vi "moveToJumperPosition-v02.vi"(0 "which manipulator":T3(ring), 1 "controls array in":refnum<vi>[](array[refnum]), 7 "Which Jumper Position to move to?":T1(ring), 9 "setStatus?":bool=TRUE, 11 "error in":errorcluster, 12 "common cluster":T2) -> (3 "control array out":refnum<vi>[](array[refnum]), 15 "error out":errorcluster)   [LabVIEW 2019]
uses:
  multipatch/controls/multipatch_common_controls_v4.ctl
  machine_vision/controls/transform_cluster_actuator.ctl
  machine_vision/coordinate model vis/transform_properties_actuators.ctl
  pipette cleaning/pressure box/cleaning_soft/controls/actuator_cluster.ctl
  pipette cleaning/pressure box/cleaning_soft/controls/actuator_type.ctl
  pipette cleaning/pressure box/cleaning_soft/controls/pressure_box_control.ctl
  pipette cleaning/pressure box/cleaning_soft/controls/pressure_box_type.ctl
  controls/NH_method.ctl
  controls/scope_motion.ctl
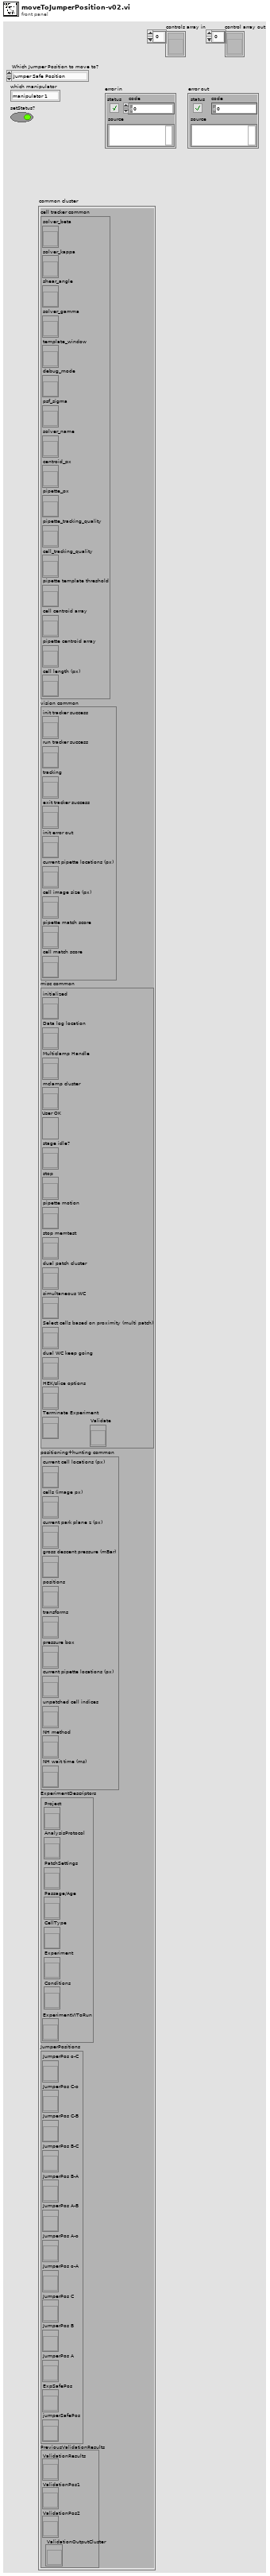
[diagram p1: front panel]
types:
  T1 = enum16{"Jumper Safe Position", "Experiment Safe Position", "Jumper Position A", "Jumper Position B", "Jumper Position C", "Jumper Position o-A", "Jumper Position A-o", "Jumper Position A-B", "Jumper Position B-A", "Jumper Position B-C", "Jumper Position C-B", "Jumper Position C-o", "Jumper Position o-C"}
  T2 = typedef "multipatch_common_controls_v4.ctl" = cluster{"cell tracker common":cluster{"solver_beta":refnum<vi>, "solver_kappa":refnum<vi>, "shear_angle":refnum<vi>, "solver_gamma":refnum<vi>, "template_window":refnum<vi>, "debug_mode":refnum<vi>, "psf_sigma":refnum<vi>, "solver_name":refnum<vi>, "centroid_px":refnum<vi>, "pipette_px":refnum<vi>, "pipette_tracking_quality":refnum<vi>, "cell_tracking_quality":refnum<vi>, "pipette template threshold":refnum<vi>, "cell centroid array":refnum<vi>, "pipette centroid array":refnum<vi>, "cell length (px)":refnum<vi>}, "vision common":cluster{"init tracker success":refnum<vi>, "run tracker success":refnum<vi>, "tracking":refnum<vi>, "exit tracker success":refnum<vi>, "init error out":refnum<vi>, "current pipette locations (px)":refnum<vi>, "cell image size (px)":refnum<vi>, "pipette match score":refnum<vi>, "cell match score":refnum<vi>}, "misc common":cluster{"initialized":refnum<vi>, "Data log location":refnum<vi>, "Multiclamp Handle":refnum<vi>, "mclamp cluster":refnum<vi>, "User OK":refnum<vi>, "stage idle?":refnum<vi>, "stop":refnum<vi>, "pipette motion":refnum<vi>, "stop memtest":refnum<vi>, "dual patch cluster":refnum<vi>, "simultaneous WC":refnum<vi>, "Select cells based on proximity (multi patch)":refnum<vi>, "dual WC keep going":refnum<vi>, "HEK/slice options":refnum<vi>, "Terminate Experiment":refnum<vi>, "Validate":refnum<vi>}, "positioning+hunting common":cluster{"current cell locations (px)":refnum<vi>, "cells (image px)":refnum<vi>, "current park plane z (px)":refnum<vi>, "gross descent pressure (mBar)":refnum<vi>, "positions":refnum<vi>, "transforms":refnum<vi>, "pressure box":refnum<vi>, "current pipette locations (px)":refnum<vi>, "unpatched cell indices":refnum<vi>, "NH method":refnum<vi>, "NH wait time (ms)":refnum<vi>}, "ExperimentDescriptors":cluster{"Project":refnum<vi>, "AnalysisProtocol":refnum<vi>, "PatchSettings":refnum<vi>, "Passage/Age":refnum<vi>, "CellType":refnum<vi>, "Experiment":refnum<vi>, "Conditions":refnum<vi>, "ExperimentVIToRun":refnum<vi>}, "JumperPositions":cluster{"JumperPos o-C":refnum<vi>, "JumperPos C-o":refnum<vi>, "JumperPos C-B":refnum<vi>, "JumperPos B-C":refnum<vi>, "JumperPos B-A":refnum<vi>, "JumperPos A-B":refnum<vi>, "JumperPos A-o":refnum<vi>, "JumperPos o-A":refnum<vi>, "JumperPos C":refnum<vi>, "JumperPos B":refnum<vi>, "JumperPos A":refnum<vi>, "ExpSafePos":refnum<vi>, "jumperSafePos":refnum<vi>}, "PreviousValidationResults":cluster{"ValidationResults":refnum<vi>, "ValidationPos1":refnum<vi>, "ValidationPos2":refnum<vi>, "ValidationOutputCluster":refnum<vi>}}
  T3 = enum16{"manipulator 1", "manipulator 2", "manipulator 3", "manipulator 4"}
  T4 = cluster{"JumperPos o-C":refnum<vi>, "JumperPos C-o":refnum<vi>, "JumperPos C-B":refnum<vi>, "JumperPos B-C":refnum<vi>, "JumperPos B-A":refnum<vi>, "JumperPos A-B":refnum<vi>, "JumperPos A-o":refnum<vi>, "JumperPos o-A":refnum<vi>, "JumperPos C":refnum<vi>, "JumperPos B":refnum<vi>, "JumperPos A":refnum<vi>, "ExpSafePos":refnum<vi>, "jumperSafePos":refnum<vi>}
  T5 = typedef "pressure_box_control.ctl" = cluster{"Pressure box COM":refnum<visa-resource-name>, "pressure box type":T6, "High pos pressure (mBar)":dbl, "Low pos pressure (mBar)":dbl, "Vacuum pressure (mBar)":dbl, "calibration":enum16{"PA_vacPump", "PA_venturi", "Neuromatics", "ilyaRig", "mightenRig"}}
  T6 = typedef "pressure_box_type.ctl" = enum16{"Neuromatics", "ProportionAir", "Demo box", "N-ProportionAir"}
  T7 = cluster{"current stage pos (steps)":refnum<vi>, "current manip 1 pos (steps)":refnum<vi>, "current manip 2 pos (steps)":refnum<vi>, "current manip 3 pos (steps)":refnum<vi>, "current manip 4 pos (steps)":refnum<vi>}
  T8 = typedef "transform_cluster_actuator.ctl" = cluster{"s":refnum<vi>, "manip 1":refnum<vi>, "manip 2":refnum<vi>, "manip 3":refnum<vi>, "manip 4":refnum<vi>}
  T9 = typedef "scope_motion.ctl" = enum16{"superSlow", "fast", "slow", "find slice speed", "slow_dualPatch"}
  T10 = typedef "transform_properties_actuators.ctl" = cluster{"theta (deg)":dbl, "X sc factor (px/step)":dbl, "Y sc factor (px/step)":dbl, "zero loc (x,y,z)":dbl[], "flip y?":bool, "flip x?":bool, "gamma (deg)":dbl, "flip z?":bool, "Z sc factor (px/step)":dbl, "actuator":T11, "safe space (steps)":i32[]}
  T11 = typedef "actuator_cluster.ctl" = cluster{"Actuator COM":refnum<visa-resource-name>, "Actuator type":T12}
  T12 = typedef "actuator_type.ctl" = enum16{"Scientifica", "Sutter", "Demo", "Off"}
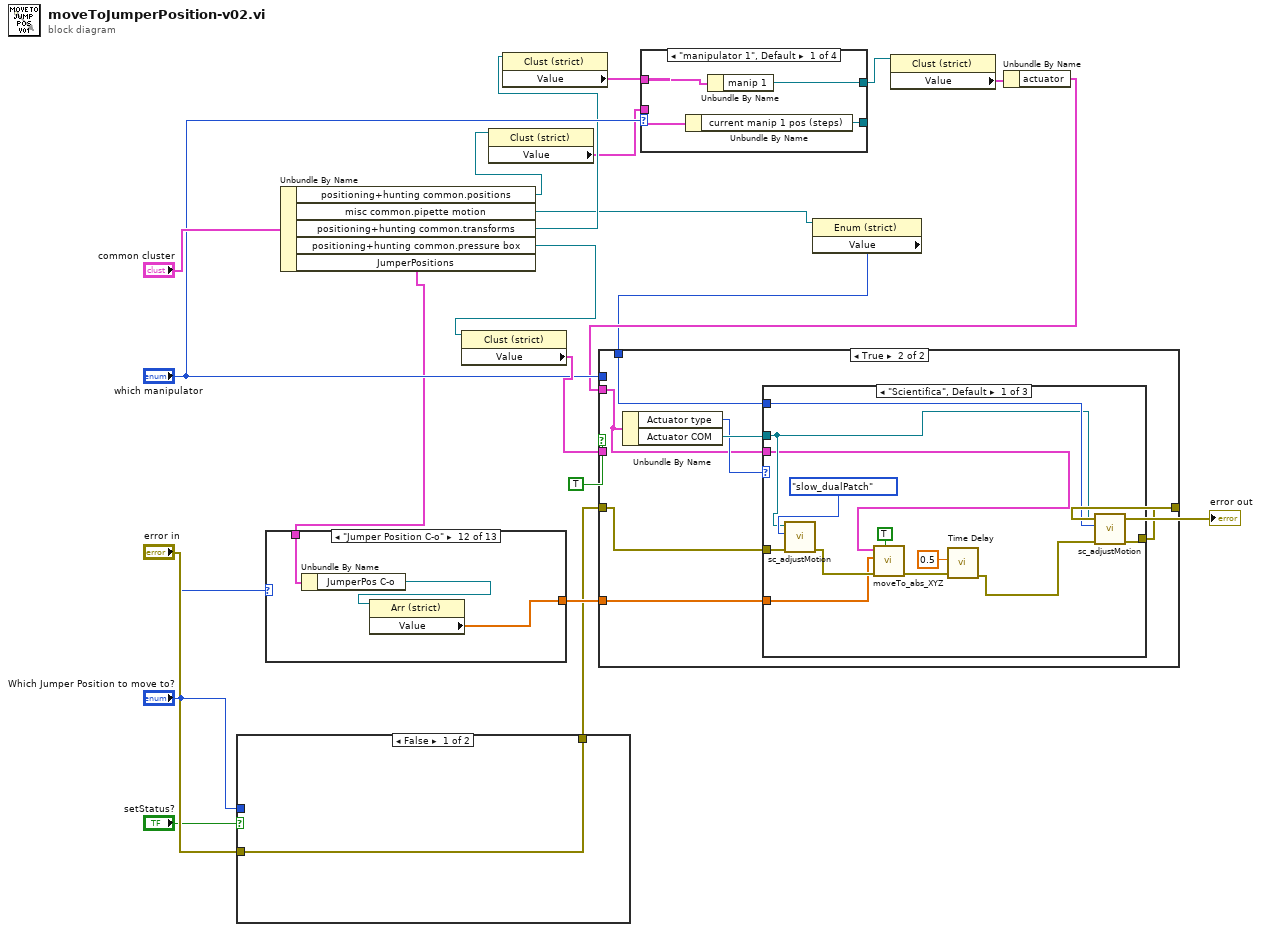
[diagram p0: block diagram]
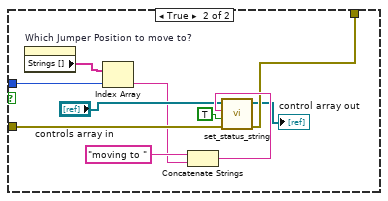
[diagram p2: hidden frame]
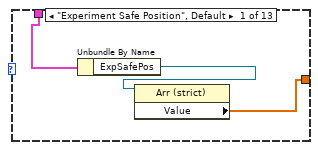
[diagram p3: hidden frame]
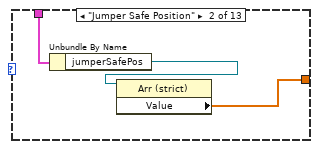
[diagram p4: hidden frame]
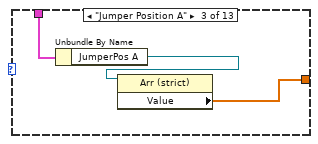
[diagram p5: hidden frame]
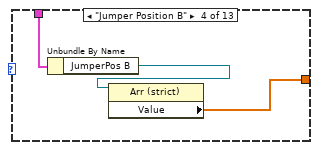
[diagram p6: hidden frame]
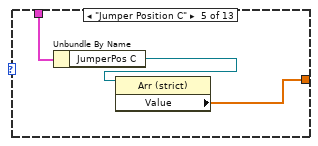
[diagram p7: hidden frame]
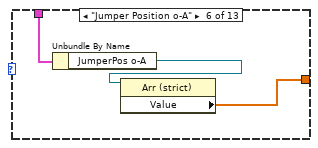
[diagram p8: hidden frame]
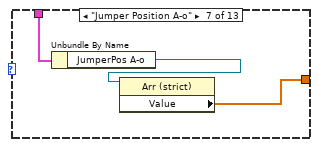
[diagram p9: hidden frame]
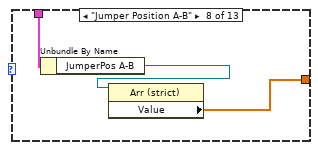
[diagram p10: hidden frame]
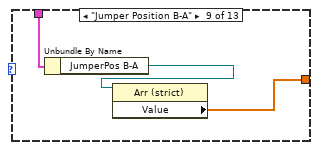
[diagram p11: hidden frame]
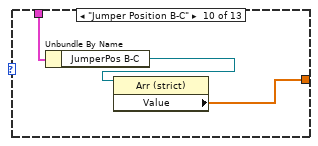
[diagram p12: hidden frame]
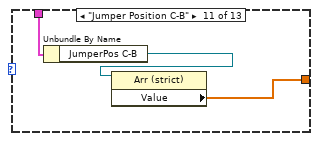
[diagram p13: hidden frame]
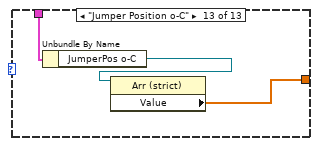
[diagram p14: hidden frame]
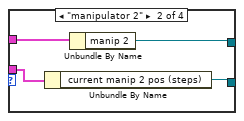
[diagram p15: hidden frame]
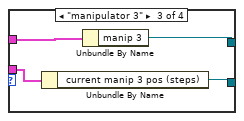
[diagram p16: hidden frame]
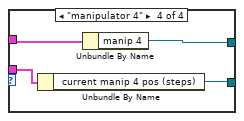
[diagram p17: hidden frame]
diagram:
  n1 = case shown="False" "setStatus?" {
    tunnel: "error in" -> [w22 w29]
    tunnel: [w22 w28] -> w3
    tunnel: "Which Jumper Position to move to?" -> [_ w24]
    frame False {
    }
    frame True {
      n2 = property on="Which Jumper Position to move to?" class="Enum (strict)"() -> ("Strings []"=w25:string[])  [unwired: 2 in, 2 out]
      n3 = Index Array(array=w25, index=w24) -> (element=w23:string)
      n4 = Concatenate Strings("moving to " ("string"), w23) -> (w31:string)
      n5 = call "set_status_string.vi"("error in"=w29, "new line?"=TRUE, "status string in"=w31, "controls array"="controls array in") -> ("error out"=w28:errorcluster, "controls array out"=→"control array out":refnum<vi>[])  [unwired: 6 in]
    }
  }
  n6 = Unbundle By Name("common cluster") -> ("positioning+hunting common.positions"=w6:refnum<vi>, "misc common.pipette motion"=w11:refnum<vi>, "positioning+hunting common.transforms"=w12:refnum<vi>, "positioning+hunting common.pressure box"=w20:refnum<vi>, "JumperPositions"=w5:T4)
  n7 = case shown="\"Jumper Position C-o\"" "Which Jumper Position to move to?" {
    tunnel: [w33 w36 w39 w42 w46 w49 w52 w55 w58 w61 w64 w67 w70] -> w7
    tunnel: w5 -> [w35 w37 w40 w43 w45 w48 w51 w54 w57 w60 w63 w66 w69]
    frame "Experiment Safe Position", Default {
      n8 = Unbundle By Name(w35) -> ("ExpSafePos"=w34:refnum<vi>)
      n9 = property class="Arr (strict)"(reference=w34) -> ("Value"=w33:dbl[])  [unwired: 1 in, 2 out]
    }
    frame "Jumper Safe Position" {
      n10 = Unbundle By Name(w37) -> ("jumperSafePos"=w38:refnum<vi>)
      n11 = property class="Arr (strict)"(reference=w38) -> ("Value"=w36:dbl[])  [unwired: 1 in, 2 out]
    }
    frame "Jumper Position A" {
      n12 = Unbundle By Name(w40) -> ("JumperPos A"=w41:refnum<vi>)
      n13 = property class="Arr (strict)"(reference=w41) -> ("Value"=w39:dbl[])  [unwired: 1 in, 2 out]
    }
    frame "Jumper Position B" {
      n14 = Unbundle By Name(w43) -> ("JumperPos B"=w44:refnum<vi>)
      n15 = property class="Arr (strict)"(reference=w44) -> ("Value"=w42:dbl[])  [unwired: 1 in, 2 out]
    }
    frame "Jumper Position C" {
      n16 = Unbundle By Name(w45) -> ("JumperPos C"=w47:refnum<vi>)
      n17 = property class="Arr (strict)"(reference=w47) -> ("Value"=w46:dbl[])  [unwired: 1 in, 2 out]
    }
    frame "Jumper Position o-A" {
      n18 = Unbundle By Name(w48) -> ("JumperPos o-A"=w50:refnum<vi>)
      n19 = property class="Arr (strict)"(reference=w50) -> ("Value"=w49:dbl[])  [unwired: 1 in, 2 out]
    }
    frame "Jumper Position A-o" {
      n20 = Unbundle By Name(w51) -> ("JumperPos A-o"=w53:refnum<vi>)
      n21 = property class="Arr (strict)"(reference=w53) -> ("Value"=w52:dbl[])  [unwired: 1 in, 2 out]
    }
    frame "Jumper Position A-B" {
      n22 = Unbundle By Name(w54) -> ("JumperPos A-B"=w56:refnum<vi>)
      n23 = property class="Arr (strict)"(reference=w56) -> ("Value"=w55:dbl[])  [unwired: 1 in, 2 out]
    }
    frame "Jumper Position B-A" {
      n24 = Unbundle By Name(w57) -> ("JumperPos B-A"=w59:refnum<vi>)
      n25 = property class="Arr (strict)"(reference=w59) -> ("Value"=w58:dbl[])  [unwired: 1 in, 2 out]
    }
    frame "Jumper Position B-C" {
      n26 = Unbundle By Name(w60) -> ("JumperPos B-C"=w62:refnum<vi>)
      n27 = property class="Arr (strict)"(reference=w62) -> ("Value"=w61:dbl[])  [unwired: 1 in, 2 out]
    }
    frame "Jumper Position C-B" {
      n28 = Unbundle By Name(w63) -> ("JumperPos C-B"=w65:refnum<vi>)
      n29 = property class="Arr (strict)"(reference=w65) -> ("Value"=w64:dbl[])  [unwired: 1 in, 2 out]
    }
    frame "Jumper Position C-o" {
      n30 = Unbundle By Name(w66) -> ("JumperPos C-o"=w68:refnum<vi>)
      n31 = property class="Arr (strict)"(reference=w68) -> ("Value"=w67:dbl[])  [unwired: 1 in, 2 out]
    }
    frame "Jumper Position o-C" {
      n32 = Unbundle By Name(w69) -> ("JumperPos o-C"=w71:refnum<vi>)
      n33 = property class="Arr (strict)"(reference=w71) -> ("Value"=w70:dbl[])  [unwired: 1 in, 2 out]
    }
  }
  n34 = property class="Clust (strict)"(reference=w20) -> ("Value"=w18:T5)  [unwired: 1 in, 2 out]
  n35 = property class="Clust (strict)"(reference=w6) -> ("Value"=w9:T7)  [unwired: 1 in, 2 out]
  n36 = property class="Clust (strict)"(reference=w12) -> ("Value"=w17:T8)  [unwired: 1 in, 2 out]
  n37 = case shown="\"manipulator 1\", Default" "which manipulator" {
    tunnel: w17 -> [w75 w79 w83 w87]
    tunnel: [w74 w78 w82 w86] -> w15
    tunnel: w9 -> [w73 w77 w81 w85]
    tunnel: [w72 w76 w80 w84] -> _
    frame "manipulator 1", Default {
      n38 = Unbundle By Name(w73) -> ("current manip 1 pos (steps)"=w72:refnum<vi>)
      n39 = Unbundle By Name(w75) -> ("manip 1"=w74:refnum<vi>)
    }
    frame "manipulator 2" {
      n40 = Unbundle By Name(w77) -> ("current manip 2 pos (steps)"=w76:refnum<vi>)
      n41 = Unbundle By Name(w79) -> ("manip 2"=w78:refnum<vi>)
    }
    frame "manipulator 3" {
      n42 = Unbundle By Name(w81) -> ("current manip 3 pos (steps)"=w80:refnum<vi>)
      n43 = Unbundle By Name(w83) -> ("manip 3"=w82:refnum<vi>)
    }
    frame "manipulator 4" {
      n44 = Unbundle By Name(w85) -> ("current manip 4 pos (steps)"=w84:refnum<vi>)
      n45 = Unbundle By Name(w87) -> ("manip 4"=w86:refnum<vi>)
    }
  }
  n46 = property class="Enum (strict)"(reference=w11) -> ("Value"=w10:T9)  [unwired: 1 in, 2 out]
  n47 = property class="Clust (strict)"(reference=w15) -> ("Value"=w14:T10)  [unwired: 1 in, 2 out]
  n48 = Unbundle By Name(w14) -> ("actuator"=w13:T11)
  n49 = case shown="True" TRUE {
    tunnel: w3 -> [w88 w93]
    tunnel: [w88 w92] -> w19
    tunnel: "which manipulator" -> [_ _]
    tunnel: w18 -> [_ _]
    tunnel: w13 -> [_ w90]
    tunnel: w10 -> [_ w91]
    tunnel: w7 -> [_ w89]
    frame False {
    }
    frame True {
      n50 = Unbundle By Name(w90) -> ("Actuator type"=w94:T12, "Actuator COM"=w95:refnum<visa-resource-name>)
      n51 = case shown="\"Scientifica\", Default" w94 {
        tunnel: w95 -> [w104 _ _]
        tunnel: [w105 w108 w109] -> w92
        tunnel: w91 -> [w107 _ _]
        tunnel: w90 -> [w103 _ _]
        tunnel: w93 -> [w97 w108 w109]
        tunnel: w89 -> [w96 _ _]
        frame "Scientifica", Default {
          n52 = call "sc_adjustMotion.vi"("error in (no error)"=w97, "motion"=scope_motion."slow_dualPatch", "VISA handle"=w104) -> ("error out"=w102:errorcluster)  [unwired: 7 in, 1 out]
          n53 = call "moveTo_abs_XYZ.vi"("blocking?"=TRUE, "error in"=w102, "XYZ location (steps)"=w96, "Actuator cluster in"=w103) -> ("error out"=w99:errorcluster)  [unwired: 6 in, 1 out]
          n54 = call "Time Delay"("error in (no error)"=w99, "Delay Time (s)"=0.5) -> ("error out"=w101:errorcluster)  [unwired: 9 in]
          n55 = call "sc_adjustMotion.vi"("error in (no error)"=w101, "motion"=w107, "VISA handle"=w104) -> ("error out"=w105:errorcluster)  [unwired: 7 in, 1 out]
        }
        frame "Sutter" {
        }
        frame "Demo" {
        }
      }
    }
  }
  "error out" <- w19
